vi "GT Get Backlash.vi"(0 "cardNum":i16, 1 "pCompDir":i32, 5 "axis":i16, 7 "pCompValue":i32, 9 "pCompChangeValue":dbl, 11 "error in (no error)":errorcluster caption="错误输入（无错误）") -> (3 "pCompDir out":i32, 4 "function return":i16, 8 "pCompValue out":i32, 10 "pCompChangeValue out":dbl, 15 "error out":errorcluster caption="错误输出")   [LabVIEW 2014, in "gts.lvlib"]
doc: "GT_API GT_GetBacklash(short cardNum,short axis,long *pCompValue,double *pCompChangeValue,long *pCompDir);"
uses:
  gts.lvlib
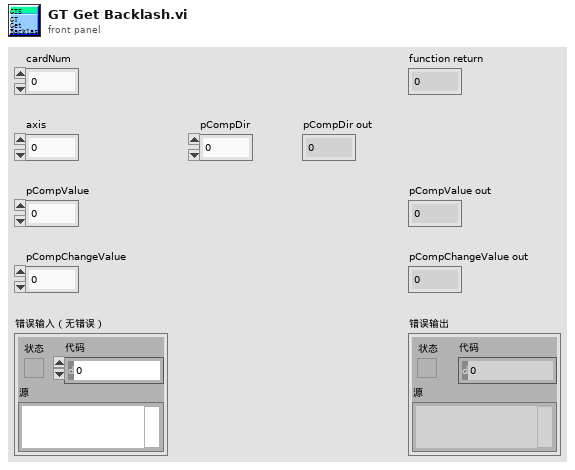
[diagram p1: front panel]
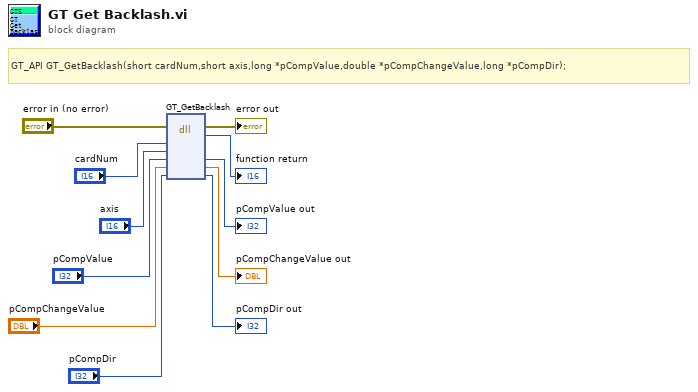
[diagram p0: block diagram]
diagram:
  # "GT_API GT_GetBacklash(short cardNum,short axis,long *pCompValue,double *pCompChangeValue,long *pCompDir);"
  n1 = dll-call lib="PTH2habs D固高科技资料GTS控制卡GTS卡18年上半年资料dllVC32bit\nmulti_cardgts.*" fn="GT_GetBacklash"(error in="error in (no error)", "cardNum"="cardNum", "axis"="axis", "pCompValue"="pCompValue", "pCompChangeValue"="pCompChangeValue", "pCompDir"="pCompDir") -> (error out=→"error out":errorcluster, →"function return":i16, "pCompValue"=→"pCompValue out":i32, "pCompChangeValue"=→"pCompChangeValue out":dbl, "pCompDir"=→"pCompDir out":i32)  [unwired: 4 in, 1 out]
